vi "Defend.vi"(11 "Maze":i32[](array[numeric])) -> (2 "Direction":T1, 3 "Defend?":bool)   [LabVIEW 2015, in "Cross.lvclass"]
uses:
  Cross.lvclass
  Type Defs/Direction Enum.ctl
  Type Defs/SB Type Defs.lvlib
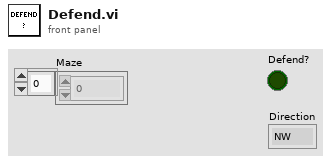
[diagram p1: front panel]
types:
  T1 = typedef "SB Type Defs.lvlib/Direction Enum.ctl" = enum16{"NW", "N", "NE", "E", "SE", "S", "SW", "W"}
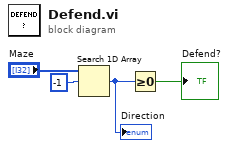
[diagram p0: block diagram]
diagram:
  n1 = Search 1D Array(1D array="Maze", element=-1) -> (index of element=w1:i32)  [unwired: 1 in]
  "Direction" <- w1
  n2 = Greater Or Equal To 0?(x=w1) -> (x >= 0?=→"Defend?":bool)
